vi "Tegam4040 -- Open4040.vi"(7 "Timeout (5000 msecs)":u32=5000, 8 "error in (no error)":errorcluster, 10 "Reset Device?":bool, 11 "VISA Resource In":refnum<visa-resource-name>) -> (0 "error out":errorcluster, 3 "Instrument Session Handle":u32 format="%x")   [LabVIEW 2010]
panel:
  out "Tegam Error Code":i32
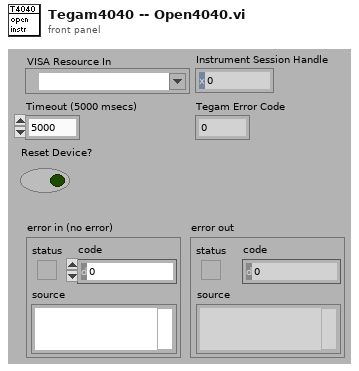
[diagram p1: front panel]
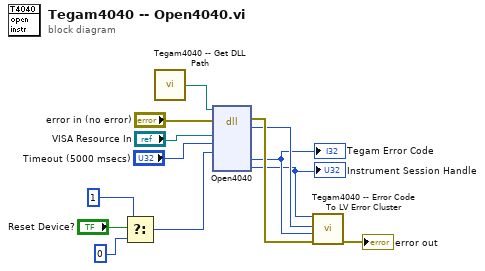
[diagram p0: block diagram]
diagram:
  n1 = Select(t=u32 1, s="Reset Device?", f=u32 0) -> (s? t:f=w1:u32)
  n2 = call "Tegam4040 -- Get DLL Path.vi"() -> ("DLL Path"=w12:path)  [unwired: 8 in]
  n3 = dll-call lib="F:/My Documents/Code/Tegam4040CDriver/release/Tegam4040CDriver.dll" fn="Open4040"(path in=w12, error in="error in (no error)", "visaResourceString"="VISA Resource In", "timeout"="Timeout (5000 msecs)", "resetDevice"=w1) -> (error out=w9:errorcluster, "visaError"=w7:i32, "tegamError"=w6:i32, "instrSessionPtr"=w5:u32)  [unwired: 6 in, 1 out]
  "Tegam Error Code" <- w6
  "Instrument Session Handle" <- w5
  n4 = call "Tegam4040 -- Error Code To LV Error Cluster.vi"("error in (no error)"=w9, "Driver Error Code"=w6, "VISA Error Code"=w7, "Instrument Session Handle"=w5) -> ("error out"=→"error out":errorcluster)  [unwired: 7 in]
